vi "Sqrt.vi"(1 "digits":i32=50, 2 "A":T1={"Array Num"=[1, 2, 3], "Decimal Index"=0, "stop"=FALSE}) -> (0 "Square Root A":T1={"Array Num"=[1, 2, 3], "Decimal Index"=0, "stop"=FALSE})   [LabVIEW 2025]
uses:
  Number.ctl
panel:
  out "?":i32
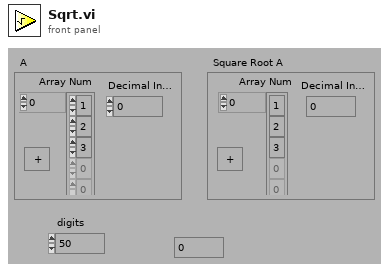
[diagram p1: front panel]
types:
  T1 = typedef "Number.ctl" = cluster{"Array Num":i8[], "Decimal Index":i32, "stop":bool}
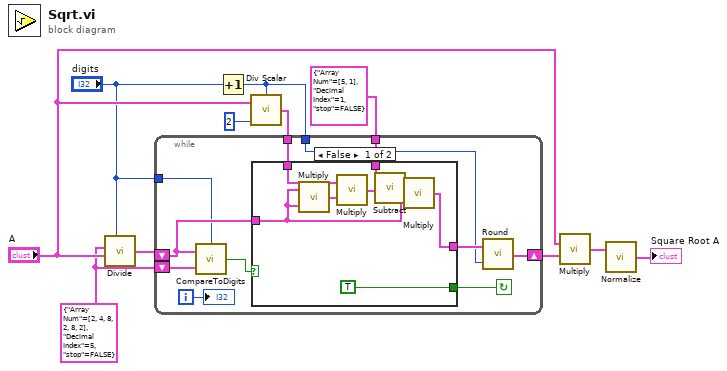
[diagram p0: block diagram]
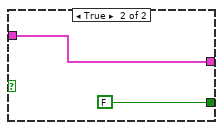
[diagram p2: hidden frame]
diagram:
  w6 = T1 {"Array Num"=[2, 4, 8, 2, 8, 2], "Decimal Index"=5, "stop"=FALSE} ("A")
  n1 = call "Divide.vi"("A"=w6, "B"="A", "digits"="digits") -> ("A/B"=w8:T1)  [unwired: 2 in]
  n2 = Increment(x="digits") -> (x+1=w2:i32)
  n3 = call "Div Scalar.vi"("Digits"=w2, "Scalar"=2, "A"="A") -> ("A / Scalar"=w10:T1)
  n4 = while {
    tunnel: T1 {"Array Num"=[5, 1], "Decimal Index"=1, "stop"=FALSE} ("A") -> [w16]
    tunnel: w10 -> [w18]
    tunnel: w2 -> [w17]
    shift-left: w6 -> [w13]
    shift-left: w8 -> [w14]
    shift-right: [w20] -> w9
    tunnel: "digits" -> [w12]
    i -> [w15]
    stop <- w21 continue-if-true
    n5 = call "CompareToDigits.vi"("Digits"=w12, "A"=w13, "A 2"=w14) -> ("Equal"=w22:bool)
    n6 = case shown="False" w22 {
      tunnel: [TRUE FALSE] -> w21
      tunnel: [w27 w31] -> w19
      tunnel: w18 -> [w28 _]
      tunnel: w16 -> [w26 _]
      tunnel: w14 -> [w23 w31]
      frame False {
        n7 = call "Multiply.vi"("B"=w23, "A"=w23) -> ("Answer"=w29:T1)
        n8 = call "Multiply.vi"("B"=w29, "A"=w28) -> ("Answer"=w25:T1)
        n9 = call "Subtract.vi"("B"=w25, "A"=w26) -> ("A-B"=w24:T1)
        n10 = call "Multiply.vi"("B"=w23, "A"=w24) -> ("Answer"=w27:T1)
      }
      frame True {
      }
    }
    n11 = call "Round.vi"("Digits"=w17, "A"=w19) -> ("A rounded to Digits"=w20:T1)
    "?" <- w15
  }
  n12 = call "Multiply.vi"("B"=w9, "A"="A") -> ("Answer"=w4:T1)
  n13 = call "Normalize.vi"("A"=w4) -> ("Normalized A"=→"Square Root A":T1)  [unwired: 1 in]
